vi "setName.vi"(8 "error in (no error)":errorcluster, 10 "Name":string, 11 "Theme.Font in":refnum<class "Theme.Font.lvclass">) -> (0 "error out":errorcluster, 3 "Theme.Font out":refnum<class "Theme.Font.lvclass">)   [LabVIEW 2017, in "Theme.lvlib" / "Theme.Font.lvclass"]
uses:
  Theme.Font.lvclass
  Theme.Font.lvclass/Theme.Font.ctl
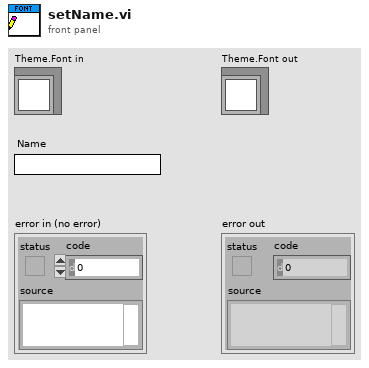
[diagram p1: front panel]
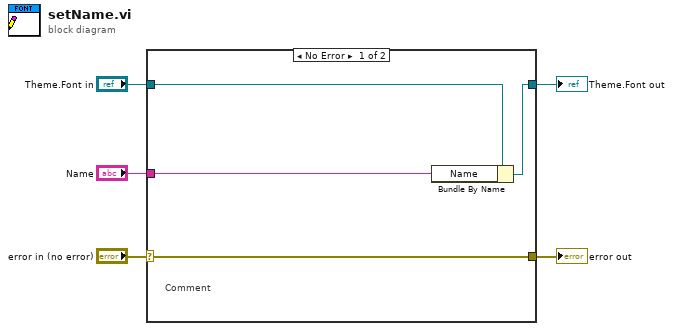
[diagram p0: block diagram]
diagram:
  n1 = case shown="No Error" "error in (no error)" {
    selector: "error in (no error)" -> [w9 w10]
    tunnel: [w9 w10] -> w4
    tunnel: [w7 w11] -> w2
    tunnel: "Theme.Font in" -> [w8 w11]
    tunnel: "Name" -> [w6 _]
    frame No Error {
      # "Comment"
      n2 = Bundle By Name(cluster=w8, "Name"=w6) -> (w7:refnum<class "Theme.Font.lvclass">)
    }
    frame Error {
    }
  }
  "error out" <- w4
  "Theme.Font out" <- w2
